vi "testString.vi"(8 "error in (no error)":errorcluster, 11 "TestCase in":refnum<class "Test Status Updater.lvclass">) -> (0 "error out":errorcluster, 3 "TestCase out":refnum<class "Test Status Updater.lvclass">)   [LabVIEW 2014, in "Test Status Updater.lvclass"]
uses:
  Test Status Updater.lvclass
  Test Status Updater.lvclass/Test Status Updater.ctl
  Core/LabVIEW CI Service/Classes/Status Updater/Status Updater.lvclass/Status Updater.ctl
  Core/LabVIEW CI Service/Classes/Status Events/Create.vi
  <vilib>/addons/_JKI Toolkits/VI Tester/TestCase.llb/TestCase.lvclass
  Core/LabVIEW CI Service/Classes/Status Updater/Status Updater.lvclass
  Core/LabVIEW CI Service/Classes/Status Events/Status Events.lvclass
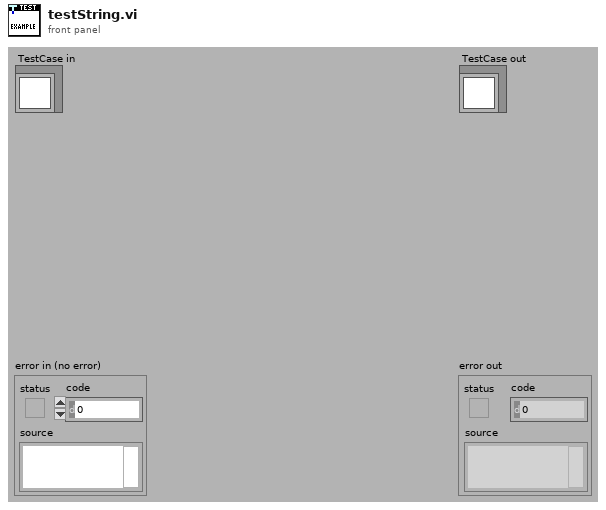
[diagram p1: front panel]
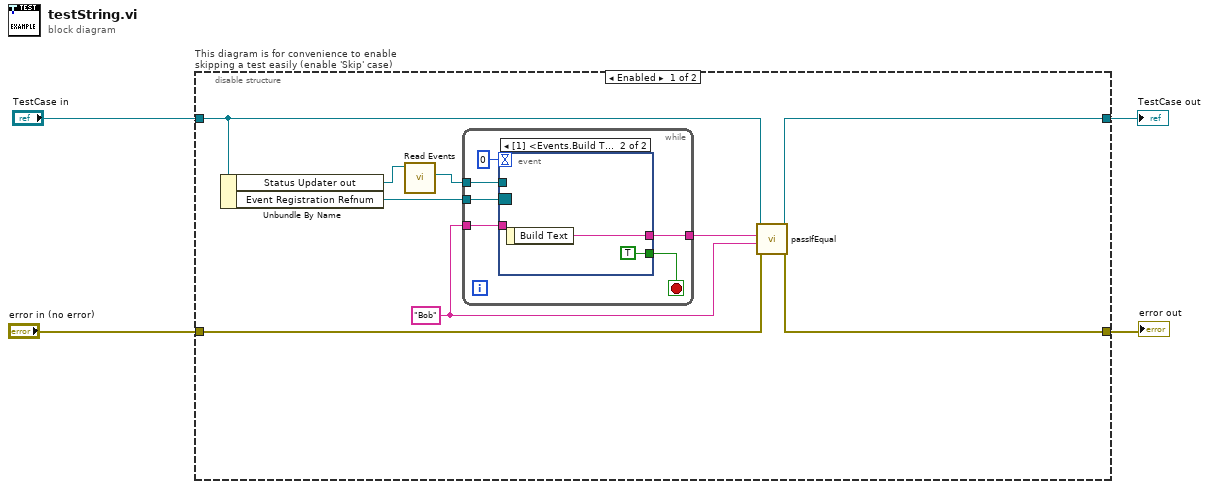
[diagram p0: block diagram]
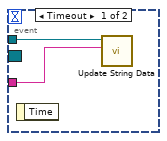
[diagram p2: hidden frame]
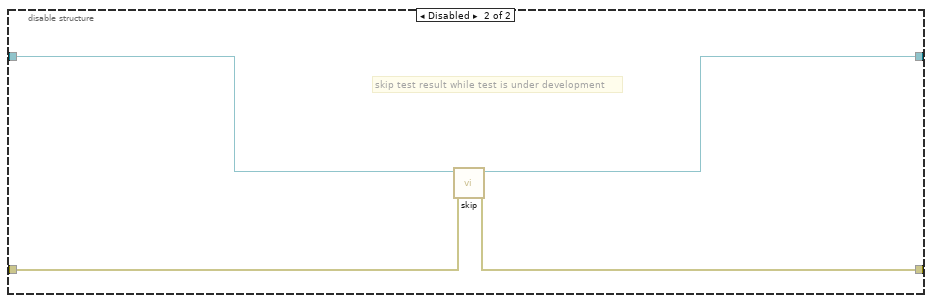
[diagram p3: hidden frame]
diagram:
  n1 = disable-structure "This diagram is for convenience to enable skipping a test easily (enable 'Skip' case)" shown="Enabled" {
    disable-tunnel: "TestCase in" -> [w10 w27]
    disable-tunnel: [w13 w25] -> w1
    disable-tunnel: [w12 w26] -> w3
    disable-tunnel: "error in (no error)" -> [w11 w24]
    frame Enabled {
      w6 = "Bob" ("String Data")
      n2 = Unbundle By Name(w10) -> ("Status Updater out"=w8:refnum<class "Status Updater.lvclass">, "Event Registration Refnum"=w9:refnum<event-registration>)
      n3 = call "Read Events.vi"("Status Updater in"=w8) -> ("Status Events"=w7:refnum<class "Status Events.lvclass">)  [unwired: 10 in]
      n4 = while {
        tunnel: w9 -> [w18]
        tunnel: w7 -> [w17]
        tunnel: w6 -> [w16]
        tunnel: [w15] -> w5
        stop <- w14 stop-if-true
        n5 = event shown="[1] <Events.Build Text>: User Event" {
          selector: w18 -> [_ _]
          dyn-events: _ -> [_ _]
          timeout: 0 -> [_ _]
          tunnel: w17 -> [w21 _]
          tunnel: [_ w23] -> w15
          tunnel: w16 -> [w20 _]
          tunnel: [_ TRUE] -> w14
          event Timeout {
            n6 = event-data() -> ()  [unwired: 1 in, 1 out]
            n7 = call "Update String Data.vi"("String Data"=w20, "Status Updater in"=w21) -> ()  [unwired: 8 in, 2 out]
          }
          event User Event {
            n8 = event-data() -> ("Build Text"=w23:string)  [unwired: 1 in]
          }
        }
      }
      n9 = call-dynamic "passIfEqual.vi"("error in (no error)"=w11, "y"=w6, "x"=w5, "TestCase in"=w10) -> ("error out"=w12:errorcluster, "TestCase out"=w13:refnum<class "Test Status Updater.lvclass">)  [unwired: 6 in]
    }
    frame Disabled {
      # "skip test result while test is under development"
      n10 = call <vilib>:"skip.vi"("error in (no error)"=w24, "TestCase in"=w27) -> ("error out"=w26:errorcluster, "TestCase out"=w25:refnum<class "Test Status Updater.lvclass">)  [unwired: 8 in]
    }
  }
  "error out" <- w3
  "TestCase out" <- w1
